vi "CfgFile Set Desc bp.vi"(8 "error in (no error)":errorcluster, 10 "bp":T1, 11 "LF2R IDE in":refnum<class "LF2R IDE.lvclass">) -> (0 "error out":errorcluster, 3 "LF2R IDE out":refnum<class "LF2R IDE.lvclass">)   [LabVIEW 2018, in "LF2R IDE.lvlib" / "LF2R IDE.lvclass"]
uses:
  LF2R IDE.lvclass
  Const UI Desc Frame bp.ctl
  Const UI Desc Property.ctl
  LF2R IDE.lvclass/LF2R IDE.ctl
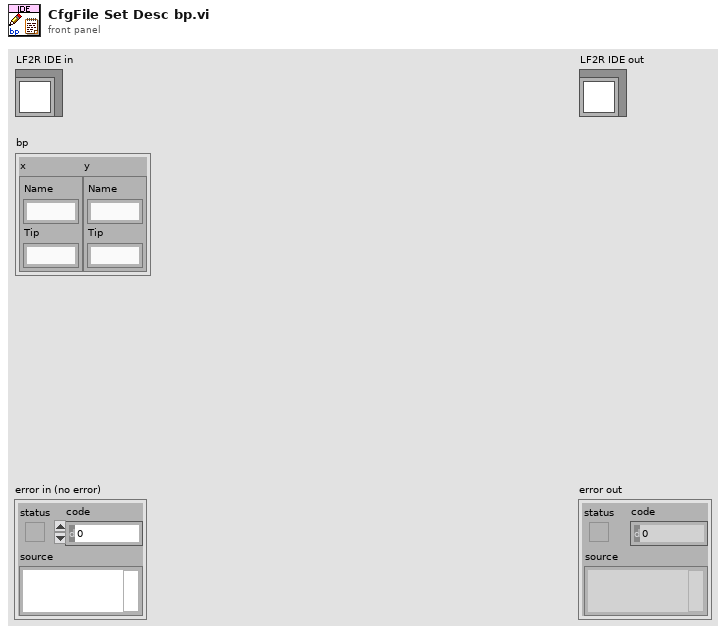
[diagram p1: front panel]
types:
  T1 = typedef "LF2R IDE.lvlib/LF2R IDE.lvclass/Const UI Desc Frame bp.ctl" = cluster{"x":T2, "y":T2}
  T2 = typedef "LF2R IDE.lvlib/LF2R IDE.lvclass/Const UI Desc Property.ctl" = cluster{"Name":string, "Tip":string}
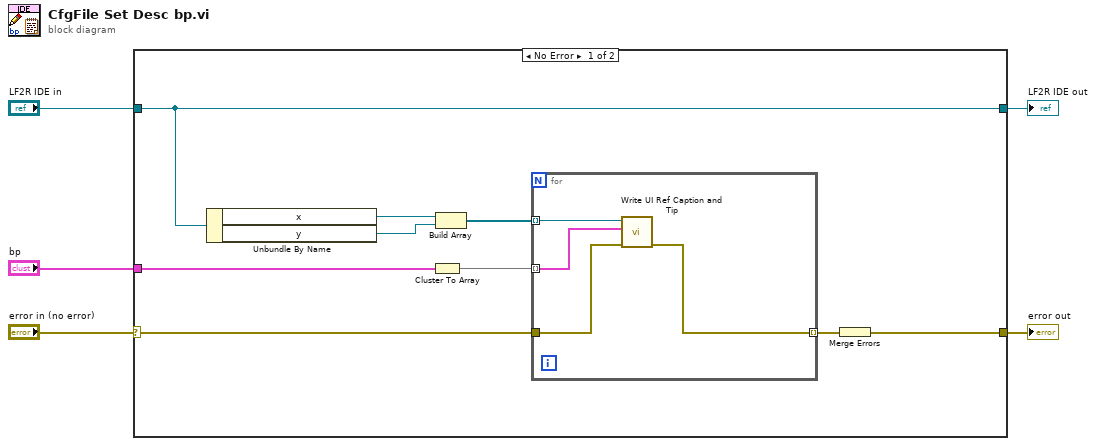
[diagram p0: block diagram]
diagram:
  n1 = case shown="No Error" "error in (no error)" {
    selector: "error in (no error)" -> [w12 w20]
    tunnel: [w10 w20] -> w4
    tunnel: [w14 w19] -> w2
    tunnel: "LF2R IDE in" -> [w14 w19]
    tunnel: "bp" -> [w7 _]
    frame No Error {
      n2 = Unbundle By Name(w14) -> ("x"=w9:refnum<vi>, "y"=w8:refnum<vi>)
      n3 = Cluster To Array(cluster=w7) -> (array=w6:T2[])
      n4 = Build Array(w9, w8) -> (w13:refnum<vi>[])
      n5 = for {
        tunnel: w13 -> [w16] mode=indexing
        tunnel: w12 -> [w18]
        tunnel: [w17] -> w11 mode=indexing
        tunnel: w6 -> [w15] mode=indexing
        n6 = call "Write UI Ref Caption and Tip.vi"("error in (no error)"=w18, "UI Property"=w15, "UI Ref"=w16) -> ("error out"=w17:errorcluster)  [unwired: 8 in]
      }
      n7 = Merge Errors(w11) -> (w10:errorcluster)
    }
    frame Error {
    }
  }
  "error out" <- w4
  "LF2R IDE out" <- w2
